vi "NoForbidden.vi"() -> ()   [LabVIEW 2014]
panel:
  in  "menu":bool
  out "current row":dbl
  out "current col":dbl
  out "whitePiece":bool
  out "blackPiece":bool
  out "black":bool[][](array[boolean])
  out "counts":dbl
  out "white":bool[][](array[boolean])
  in  "resume":bool caption="restart"
  out "status":bool
  out "?":bool
  in  "redo":bool
  out "?":bool
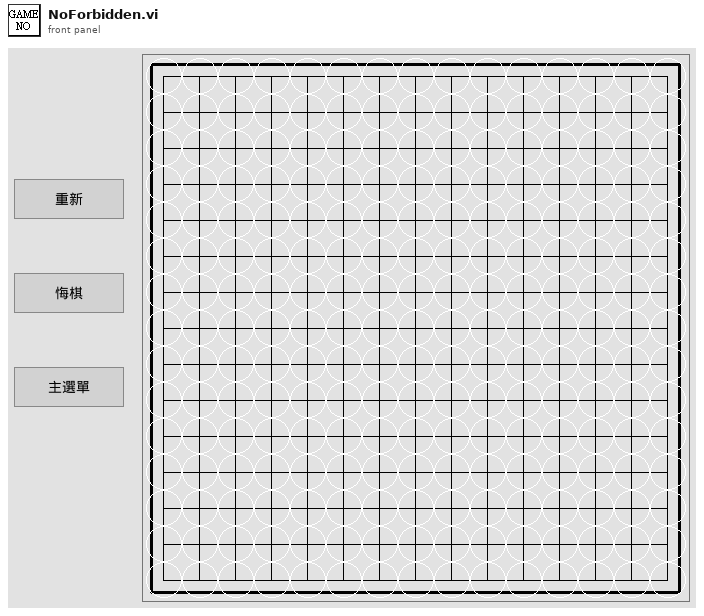
[diagram p1: front panel]
types:
  T1 = typedef "LVPoint32TypeDef.ctl" = cluster{"Horizontal":i32, "Vertical":i32}
  T2 = cluster{"Numeric Control":dbl, "Numeric Control":dbl}
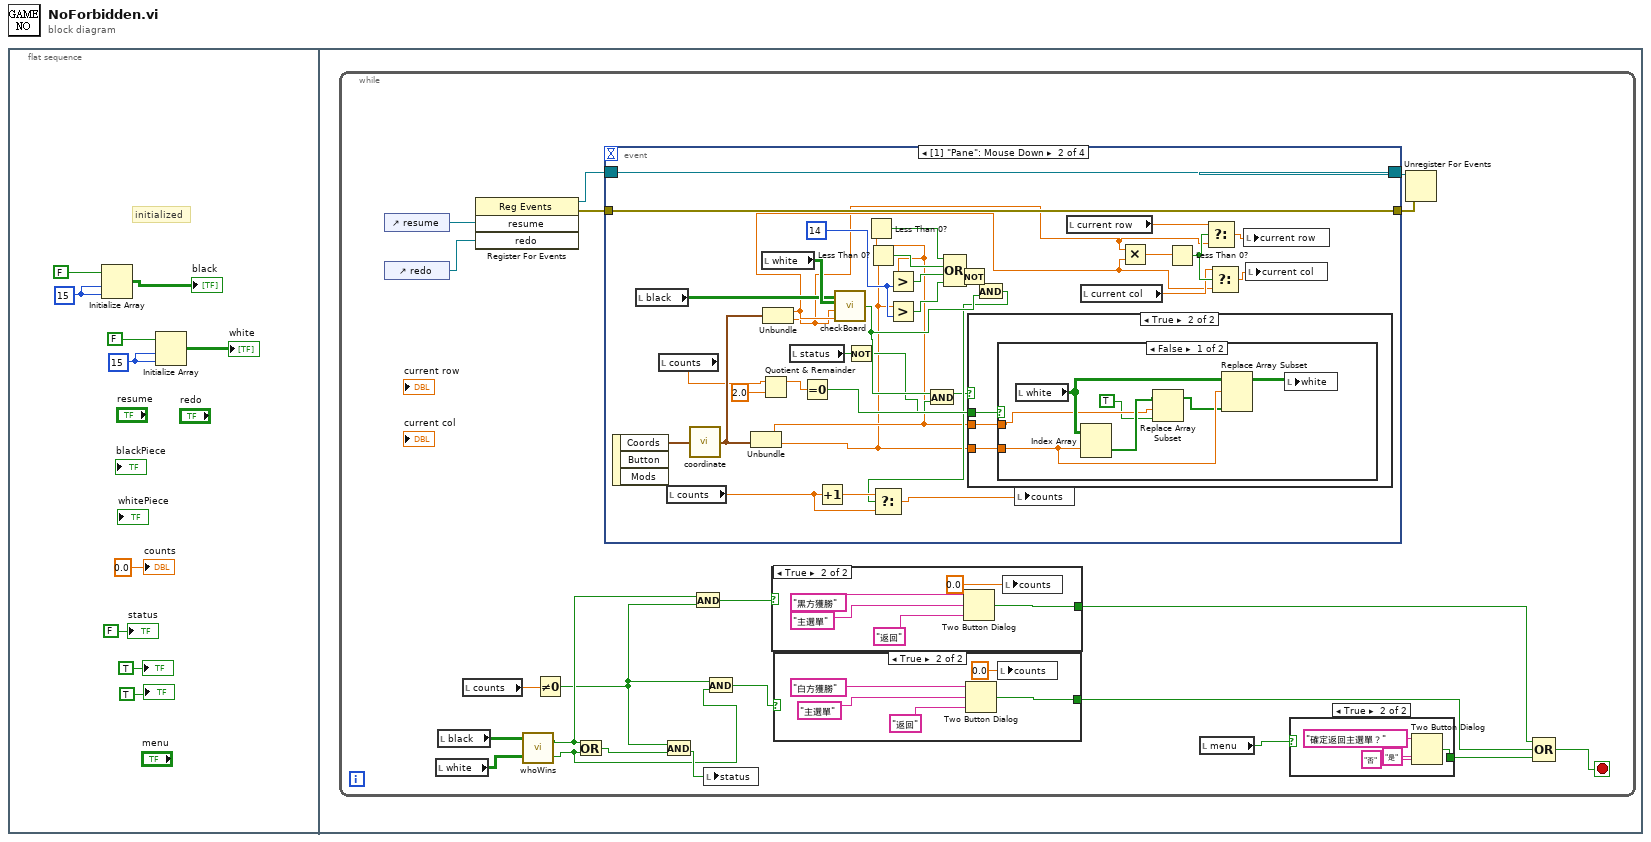
[diagram p0: block diagram]
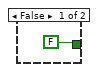
[diagram p2: hidden frame]
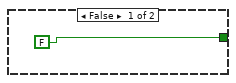
[diagram p3: hidden frame]
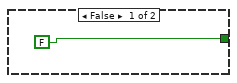
[diagram p4: hidden frame]
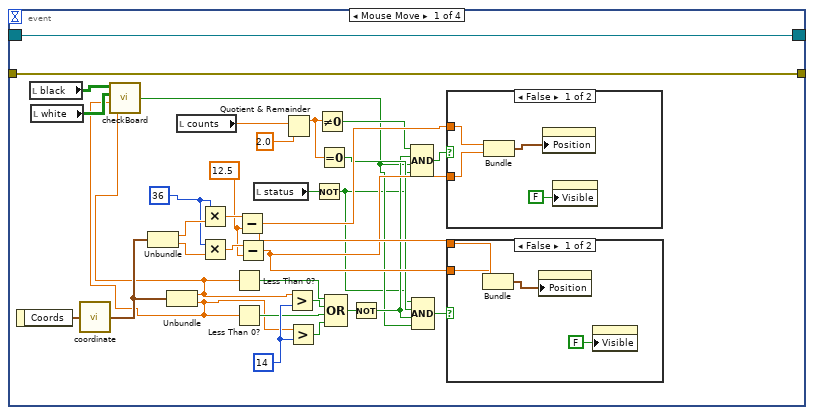
[diagram p5: hidden frame]
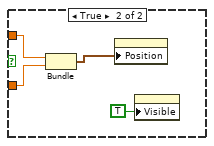
[diagram p6: hidden frame]
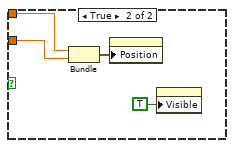
[diagram p7: hidden frame]
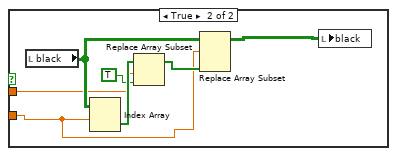
[diagram p9: hidden frame]
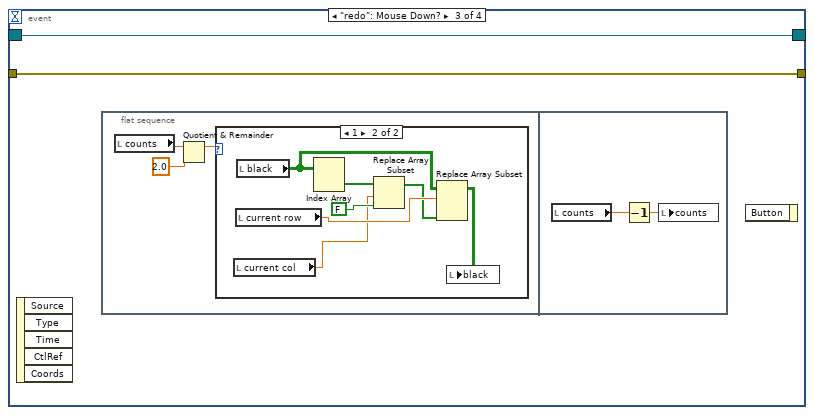
[diagram p10: hidden frame]
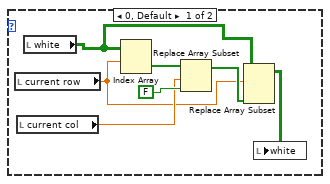
[diagram p11: hidden frame]
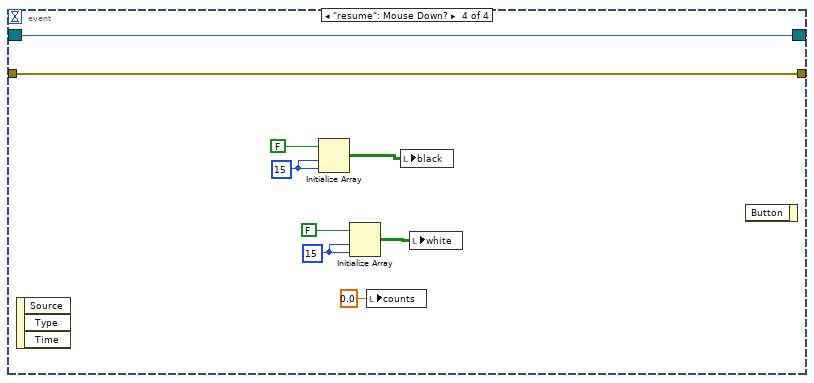
[diagram p12: hidden frame]
diagram:
  n1 = flat-sequence {
    frame #0 {
      w9 = 15
      w6 = 15
      # "initialized"
      n2 = Initialize Array(FALSE, w6, w6) -> (→"black":bool[][])
      n3 = Initialize Array(FALSE, w9, w9) -> (→"white":bool[][])
      "counts" <- 0.0 ("Numeric Indicator")
      "status" <- FALSE ("status")
      "?" <- TRUE
      "?" <- TRUE
    }
    frame #1 {
      n4 = while {
        stop <- w17 stop-if-true
        n5 = control-ref of="resume"() -> (w27:refnum<vi>)
        n6 = control-ref of="redo"() -> (w23:refnum<vi>)
        n7 = local read "white"() -> (w20:bool[][])
        n8 = local read "black"() -> (w21:bool[][])
        n9 = local read "counts"() -> (w25:dbl)
        n10 = register-events(w27, w23) -> (reference out=w29:refnum<event-registration>, error out=w31:errorcluster)  [unwired: 2 in]
        n11 = call "whoWins.vi"("white"=w20, "black"=w21) -> ("wWins"=w13:bool, "bWins"=w15:bool)
        n12 = Not Equal To 0?(x=w25) -> (x != 0?=w11:bool)
        n13 = Or(x=w15, y=w13) -> (x .or. y?=w26:bool)
        n14 = event shown="[1] \"Pane\": Mouse Down" {
          selector: w29 -> [w81 w132 w151 w178]
          dyn-events: [w81 w132 w151 w178] -> w28
          timeout: _ -> [_ _ _ _]
          tunnel: w31 -> [w80 w131 w150 w177]
          tunnel: [w80 w131 w150 w177] -> w30
          event Mouse Move {
            w71 = 14
            w73 = 12.5
            w76 = 36
            n15 = event-data() -> ("Coords"=w79:T1)  [unwired: 1 in]
            n16 = local read "black"() -> (w55:bool[][])
            n17 = local read "white"() -> (w54:bool[][])
            n18 = call "coordinate.vi"("Cluster"=w79) -> ("output cluster"=w72:T2)
            n19 = Unbundle(w72) -> ("Numeric Control"=w78:dbl, "Numeric Control"=w77:dbl)
            n20 = Unbundle(w72) -> ("Numeric Control"=w53:dbl, "Numeric Control"=w52:dbl)
            n21 = call "checkBoard.vi"("column"=w53, "row"=w52, "white"=w54, "black"=w55) -> ("element"=w51:bool)
            n22 = local read "counts"() -> (w64:dbl)
            n23 = Multiply(x=w76, y=w78) -> (x*y=w75:dbl)
            n24 = Multiply(x=w76, y=w77) -> (x*y=w74:dbl)
            n25 = Less Than 0?(x=w53) -> (x < 0?=w70:bool)
            n26 = Less Than 0?(x=w52) -> (x < 0?=w68:bool)
            n27 = Subtract(x=w75, y=w73) -> (x-y=w66:dbl)
            n28 = Subtract(x=w74, y=w73) -> (x-y=w65:dbl)
            n29 = local read "status"() -> (w50:bool)
            n30 = Quotient & Remainder(x=w64, y=2.0) -> (x-y*floor(x/y)=w58:dbl)  [unwired: 1 out]
            n31 = Greater?(x=w53, y=w71) -> (0:w69:bool)
            n32 = Greater?(x=w52, y=w71) -> (0:w67:bool)
            n33 = Not(x=w50) -> (.not. x?=w49:bool)
            n34 = Not Equal To 0?(x=w58) -> (x != 0?=w59:bool)
            n35 = Equal To 0?(x=w58) -> (x = 0?=w57:bool)
            n36 = Compound Arithmetic op=OR(w70, w69, w68, w67) -> (w60:bool)
            n37 = Not(x=w60) -> (.not. x?=w56:bool)
            n38 = Compound Arithmetic op=AND(w59, w56, w51, w49) -> (w62:bool)
            n39 = Compound Arithmetic op=AND(w49, w57, w56, w51) -> (w61:bool)
            n40 = case shown="False" w62 {
              tunnel: w66 -> [w85 w88]
              tunnel: w65 -> [w84 w87]
              frame False {
                n41 = Bundle(w85, w84) -> (w83:cluster{dbl, dbl})  [unwired: 1 in]
                n42 = property class="Bool (strict)"("Position"=w83) -> ()  [unwired: 2 in, 2 out]
                n43 = property class="Bool (strict)"("Visible"=FALSE) -> ()  [unwired: 2 in, 2 out]
              }
              frame True {
                n44 = Bundle(w88, w87) -> (w86:cluster{dbl, dbl})  [unwired: 1 in]
                n45 = property class="Bool (strict)"("Position"=w86) -> ()  [unwired: 2 in, 2 out]
                n46 = property class="Bool (strict)"("Visible"=TRUE) -> ()  [unwired: 2 in, 2 out]
              }
            }
            n47 = case shown="False" w61 {
              tunnel: w66 -> [w92 w97]
              tunnel: w65 -> [w91 w96]
              frame False {
                n48 = Bundle(w92, w91) -> (w93:cluster{dbl, dbl})  [unwired: 1 in]
                n49 = property class="Bool (strict)"("Position"=w93) -> ()  [unwired: 2 in, 2 out]
                n50 = property class="Bool (strict)"("Visible"=FALSE) -> ()  [unwired: 2 in, 2 out]
              }
              frame True {
                n51 = Bundle(w97, w96) -> (w95:cluster{dbl, dbl})  [unwired: 1 in]
                n52 = property class="Bool (strict)"("Position"=w95) -> ()  [unwired: 2 in, 2 out]
                n53 = property class="Bool (strict)"("Visible"=TRUE) -> ()  [unwired: 2 in, 2 out]
              }
            }
          }
          event Mouse Down {
            w119 = 14
            n54 = event-data() -> ("Coords"=w130:T1)  [unwired: 1 in, 2 out]
            n55 = local read "black"() -> (w124:bool[][])
            n56 = local read "counts"() -> (w128:dbl)
            n57 = local read "counts"() -> (w122:dbl)
            n58 = call "coordinate.vi"("Cluster"=w130) -> ("output cluster"=w129:T2)
            n59 = Unbundle(w129) -> ("Numeric Control"=w107:dbl, "Numeric Control"=w106:dbl)
            n60 = Quotient & Remainder(x=w128, y=2.0) -> (x-y*floor(x/y)=w126:dbl)  [unwired: 1 out]
            n61 = local read "white"() -> (w125:bool[][])
            n62 = Unbundle(w129) -> ("Numeric Control"=w100:dbl, "Numeric Control"=w99:dbl)
            n63 = local read "status"() -> (w109:bool)
            n64 = Equal To 0?(x=w126) -> (x = 0?=w123:bool)
            n65 = Increment(x=w122) -> (x+1=w120:dbl)
            n66 = call "checkBoard.vi"("column"=w100, "row"=w99, "white"=w125, "black"=w124) -> ("element"=w113:bool)
            n67 = Not(x=w109) -> (.not. x?=w108:bool)
            n68 = Less Than 0?(x=w107) -> (x < 0?=w118:bool)
            n69 = Less Than 0?(x=w106) -> (x < 0?=w117:bool)
            n70 = Greater?(x=w107, y=w119) -> (0:w116:bool)
            n71 = Greater?(x=w106, y=w119) -> (0:w115:bool)
            n72 = And(x=w113, y=w108) -> (x .and. y?=w110:bool)
            n73 = Compound Arithmetic op=OR(w118, w117, w116, w115) -> (w114:bool)
            n74 = Not(x=w114) -> (.not. x?=w111:bool)
            n75 = case shown="True" w110 {
              tunnel: w107 -> [_ w135]
              tunnel: w106 -> [_ w134]
              tunnel: w123 -> [_ w133]
              frame False {
              }
              frame True {
                n76 = case shown="False" w133 {
                  tunnel: w135 -> [w138 w144]
                  tunnel: w134 -> [w140 w143]
                  frame False {
                    n77 = local read "white"() -> (w142:bool[][])
                    n78 = Index Array(array=w142, index (row)=w140) -> (element=w139:bool[])  [unwired: 1 in]
                    n79 = Replace Array Subset(array=w139, new element=TRUE, index=w138) -> (w136:bool[])
                    n80 = Replace Array Subset(array=w142, new element=w136, index (row)=w140) -> (w141:bool[][])  [unwired: 1 in]
                    n81 = local write "white"(w141) -> ()
                  }
                  frame True {
                    n82 = local read "black"() -> (w146:bool[][])
                    n83 = Index Array(array=w146, index (row)=w143) -> (element=w149:bool[])  [unwired: 1 in]
                    n84 = Replace Array Subset(array=w149, new element=TRUE, index=w144) -> (w147:bool[])
                    n85 = Replace Array Subset(array=w146, new element=w147, index (row)=w143) -> (w145:bool[][])  [unwired: 1 in]
                    n86 = local write "black"(w145) -> ()
                  }
                }
              }
            }
            n87 = And(x=w111, y=w113) -> (x .and. y?=w112:bool)
            n88 = Select(t=w120, s=w112, f=w122) -> (s? t:f=w121:dbl)
            n89 = local write "counts"(w121) -> ()
            n90 = local read "current row"() -> (w104:dbl)
            n91 = local read "current col"() -> (w101:dbl)
            n92 = Multiply(x=w99, y=w100) -> (x*y=w105:dbl)
            n93 = Less Than 0?(x=w105) -> (x < 0?=w102:bool)
            n94 = Select(t=w104, s=w102, f=w99) -> (s? t:f=w103:dbl)
            n95 = Select(t=w101, s=w102, f=w100) -> (s? t:f=w98:dbl)
            n96 = local write "current row"(w103) -> ()
            n97 = local write "current col"(w98) -> ()
          }
          event "redo": Mouse Down? {
            n98 = event-data() -> ()  [unwired: 1 in, 5 out]
            n99 = flat-sequence {
              frame #0 {
                n100 = local read "counts"() -> (w154:dbl)
                n101 = Quotient & Remainder(x=w154, y=2.0) -> (x-y*floor(x/y)=w152:dbl)  [unwired: 1 out]
                n102 = case shown="1" w152 {
                  frame 0, Default {
                    n103 = local read "current row"() -> (w157:dbl)
                    n104 = local read "current col"() -> (w159:dbl)
                    n105 = local read "white"() -> (w156:bool[][])
                    n106 = Index Array(array=w156, index (row)=w157) -> (element=w161:bool[])  [unwired: 1 in]
                    n107 = Replace Array Subset(array=w161, new element=FALSE, index=w159) -> (w158:bool[])
                    n108 = Replace Array Subset(array=w156, new element=w158, index (row)=w157) -> (w155:bool[][])  [unwired: 1 in]
                    n109 = local write "white"(w155) -> ()
                  }
                  frame 1 {
                    n110 = local read "current col"() -> (w165:dbl)
                    n111 = local read "current row"() -> (w166:dbl)
                    n112 = local read "black"() -> (w164:bool[][])
                    n113 = Index Array(array=w164) -> (element=w168:bool[])  [unwired: 2 in]
                    n114 = Replace Array Subset(array=w168, new element=FALSE, index=w165) -> (w162:bool[])
                    n115 = Replace Array Subset(array=w164, new element=w162, index (row)=w166) -> (w163:bool[][])  [unwired: 1 in]
                    n116 = local write "black"(w163) -> ()
                  }
                }
              }
              frame #1 {
                n117 = local read "counts"() -> (w170:dbl)
                n118 = Decrement(x=w170) -> (x-1=w169:dbl)
                n119 = local write "counts"(w169) -> ()
              }
            }
            n120 = event-data() -> ()  [unwired: 2 in, 1 out]
          }
          event "resume": Mouse Down? {
            w173 = 15
            w176 = 15
            n121 = event-data() -> ()  [unwired: 1 in, 3 out]
            n122 = Initialize Array(FALSE, w173, w173) -> (w171:bool[][])
            n123 = Initialize Array(FALSE, w176, w176) -> (w174:bool[][])
            n124 = local write "counts"(0.0 ("counts")) -> ()
            n125 = local write "black"(w171) -> ()
            n126 = local write "white"(w174) -> ()
            n127 = event-data() -> ()  [unwired: 2 in, 1 out]
          }
        }
        n128 = And(x=w11, y=w26) -> (x .and. y?=w24:bool)
        n129 = And(x=w15, y=w11) -> (x .and. y?=w14:bool)
        n130 = local write "status"(w24) -> ()
        n131 = And(x=w11, y=w13) -> (x .and. y?=w12:bool)
        n132 = case shown="True" w14 {
          tunnel: [FALSE w45] -> w19
          frame False {
          }
          frame True {
            n133 = Two Button Dialog(message="黑方獲勝", 1:"返回", 2:"主選單") -> (T button?=w45:bool)
            n134 = local write "counts"(0.0 ("counts")) -> ()
          }
        }
        n135 = case shown="True" w12 {
          tunnel: [FALSE w39] -> w18
          frame False {
          }
          frame True {
            n136 = Two Button Dialog(message="白方獲勝", 1:"返回", 2:"主選單") -> (T button?=w39:bool)
            n137 = local write "counts"(0.0 ("counts")) -> ()
          }
        }
        n138 = local read "menu"() -> (w22:bool)
        n139 = case shown="True" w22 {
          tunnel: [FALSE w35] -> w16
          frame False {
          }
          frame True {
            n140 = Two Button Dialog(message="確定返回主選單？", 1:"否" ("F button name (\"Cancel\")"), 2:"是" ("T button name (\"OK\")")) -> (T button?=w35:bool)
          }
        }
        n141 = Unregister For Events(event registration refnum=w28, error in=w30) -> ()  [unwired: 1 out]
        n142 = Compound Arithmetic op=OR(w19, w18, w16) -> (w17:bool)
      }
    }
  }
